vi "Teleop.vi"(0 "Call Context":T2, 1 "Match Info":T1={"Autonomous Elapsed Seconds"=0.0, "TeleOp Elapsed Seconds"=0.0, "Disabled Elapsed Seconds"=0.0, "Visited Autonomous"=FALSE, "Visited TeleOp"=FALSE, "Visited Disabled"=FALSE, "Autonomous Settings"={"Autonomous Style"=enum."Independent", "VI Refnum"=refnum}}) -> ()   [LabVIEW 2017]
doc: "This VI is called for each TeleOp packet received from the DS where the robot is not disabled. It is often used to read from the joysticks and update I/O or to update setpoints for timed control loops. It should complete and return within 20 milliseconds or it may miss DS packets."
uses:
  <vilib>/Rock Robotics/WPI/DriverStation/WPI_DriverStationDerivedRobotMode.ctl
  <vilib>/Rock Robotics/WPI/DriverStation/WPI_DriverStationMatch Info.ctl
  <vilib>/Rock Robotics/WPI/Utilities/WPI_GetSetVariantRefNum.vi
  <vilib>/Rock Robotics/Network Tables/NT Write Boolean Array.vi
  <vilib>/Rock Robotics/Network Tables/NT Write Numeric Array.vi
  <vilib>/Rock Robotics/Network Tables/NT Read Boolean.vi
  <vilib>/Rock Robotics/Network Tables/NT Read Number.vi
panel:
  out "Sample Slider 0":dbl(slide) scale=0.0..5.0
  out "Sample Boolean 1":bool
  out "Sample Boolean 0":bool
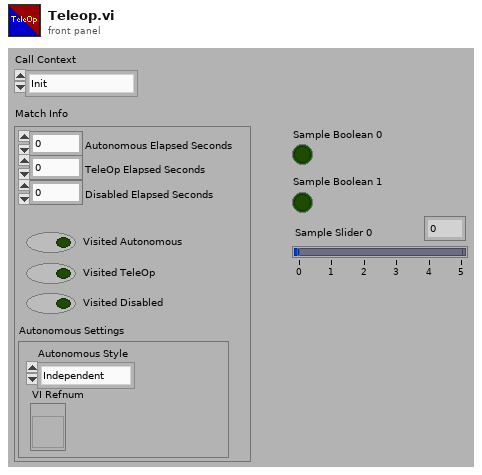
[diagram p1: front panel]
types:
  T1 = typedef "WPI_DriverStationMatch Info.ctl" = cluster{"Autonomous Elapsed Seconds":dbl, "TeleOp Elapsed Seconds":dbl, "Disabled Elapsed Seconds":dbl, "Visited Autonomous":bool, "Visited TeleOp":bool, "Visited Disabled":bool, "Autonomous Settings":cluster{"Autonomous Style":enum16{"Iterative", "Independent"}, "VI Refnum":refnum<vi>}}
  T2 = typedef "WPI_DriverStationDerivedRobotMode.ctl" = enum16{"Init", "Execute", "Stop"}
  T3 = typedef "WPI_JoystickDevRef.ctl" = cluster{"Device":T4}
  T4 = typedef "WPI_JoystickDeviceEnum.ctl" = enum16{"USB 0", "USB 1", "USB 2", "USB 3", "USB 4", "USB 5"}
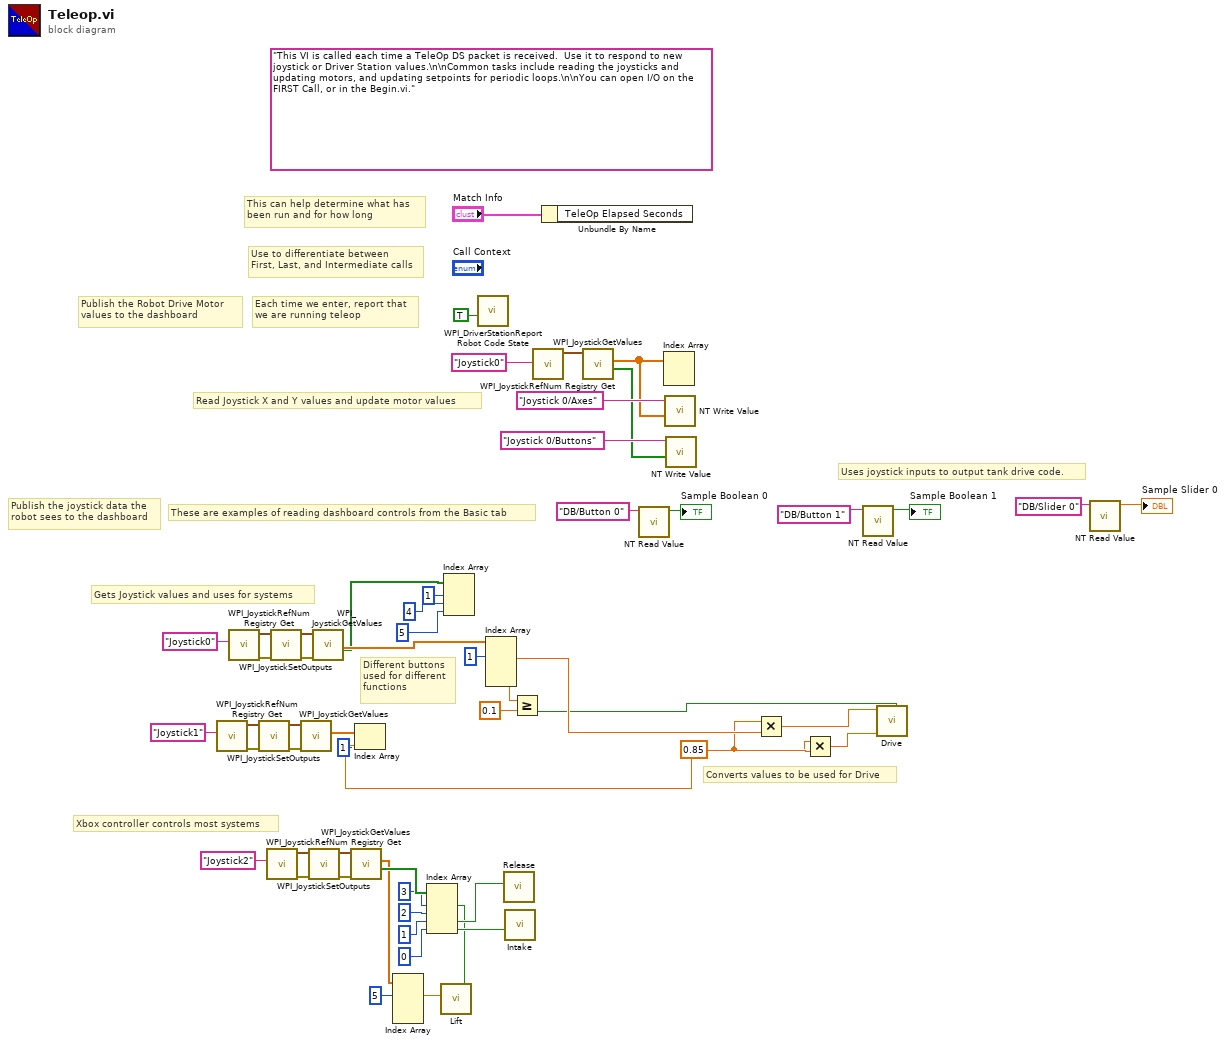
[diagram p0: block diagram]
diagram:
  w25 = 0.85
  (unwired) "This VI is called each time a TeleOp DS packet is received.  Use it to respond to new joystick or Driver Station values.\n\nCommon tasks include reading the joysticks and updating motors, and updating setpoints for periodic loops.\n\nYou can open I/O on the FIRST Call, or in the Begin.vi."
  # "Xbox controller controls most systems"
  # "Converts values to be used for Drive"
  # "Different buttons\nused for different\nfunctions"
  # "Gets Joystick values and uses for systems"
  # "Uses joystick inputs to output tank drive code."
  # "These are examples of reading dashboard controls from the Basic tab"
  # "Publish the Robot Drive Motor\nvalues to the dashboard"
  # "Publish the joystick data the\nrobot sees to the dashboard"
  # "Each time we enter, report that\nwe are running teleop"
  # "Use to differentiate between\nFirst, Last, and Intermediate calls"
  # "This can help determine what has\nbeen run and for how long"
  # "Read Joystick X and Y values and update motor values"
  n1 = call <vilib>:"WPI_JoystickRefNum Registry Get.vi"("refnum name"="Joystick1") -> ("error out"=w32:errorcluster, "JoystickDevRef"=w30:T3)  [unwired: 1 in, 8 out]
  n2 = call <vilib>:"WPI_JoystickRefNum Registry Get.vi"("refnum name"="Joystick0") -> ("error out"=w35:errorcluster, "JoystickDevRef"=w37:T3)  [unwired: 1 in, 8 out]
  n3 = call <vilib>:"WPI_JoystickSetOutputs.vi"("error in (no error)"=w32, "JoystickDevRef"=w30) -> ("error out"=w33:errorcluster, "JoystickDevRef"=w31:T3)  [unwired: 8 in]
  n4 = call <vilib>:"WPI_JoystickRefNum Registry Get.vi"("refnum name"="Joystick2") -> ("error out"=w15:errorcluster, "JoystickDevRef"=w17:T3)  [unwired: 1 in, 8 out]
  n5 = call <vilib>:"WPI_JoystickSetOutputs.vi"("error in (no error)"=w35, "JoystickDevRef"=w37) -> ("error out"=w34:errorcluster, "JoystickDevRef"=w36:T3)  [unwired: 8 in]
  n6 = call <vilib>:"WPI_JoystickGetValues.vi"("error in (no error)"=w33, "JoystickDevRef"=w31) -> ("Axes"=w28:dbl[])  [unwired: 5 in, 4 out]
  n7 = call <vilib>:"WPI_JoystickSetOutputs.vi"("error in (no error)"=w15, "JoystickDevRef"=w17) -> ("error out"=w14:errorcluster, "JoystickDevRef"=w16:T3)  [unwired: 8 in]
  n8 = call <vilib>:"WPI_JoystickGetValues.vi"("error in (no error)"=w34, "JoystickDevRef"=w36) -> ("Buttons"=w19:bool[], "Axes"=w42:dbl[])  [unwired: 5 in, 3 out]
  n9 = call <vilib>:"WPI_JoystickGetValues.vi"("error in (no error)"=w14, "JoystickDevRef"=w16) -> ("Buttons"=w13:bool[], "Axes"=w8:dbl[])  [unwired: 5 in, 3 out]
  n10 = Index Array(array=w28, index=1) -> (element=w26:dbl)
  n11 = Index Array(array=w8, index #1=5 ("index")) -> (element #1=w4:dbl)  [unwired: 3 in, 3 out]
  n12 = Index Array(array=w13, index #1=3 ("index"), index #2=2 ("index"), index #3=1 ("index"), index #4=0 ("index")) -> (element #1=w1:bool, element #3=w2:bool, element #4=w3:bool)  [unwired: 1 out]
  n13 = call "Lift.vi"("Half Effort"=w1, "Effort"=w4) -> ()  [unwired: 10 in]
  n14 = Index Array(array=w19, index #1=1 ("index"), index #2=4 ("index"), index #3=5 ("index")) -> ()  [unwired: 3 out]
  n15 = call <vilib>:"WPI_DriverStationReport Robot Code State.vi"("TeleOp"=TRUE ("Autonomous")) -> ()  [unwired: 10 in, 1 out]
  n16 = Index Array(array=w42, index #1=1 ("index")) -> (element #1=w27:dbl, element #3=w40:dbl)  [unwired: 3 in, 2 out]
  n17 = call "Release.vi"("Releasebuttonpressed?"=w2) -> ()  [unwired: 11 in]
  n18 = call "Intake.vi"("Intake?"=w3) -> ()  [unwired: 11 in]
  n19 = Greater Or Equal?(x=w40, y=0.1) -> (x >= y?=w22:bool)
  n20 = call <vilib>:"WPI_JoystickRefNum Registry Get.vi"("refnum name"="Joystick0") -> ("JoystickDevRef"=w54:T3)  [unwired: 1 in, 9 out]
  n21 = Unbundle By Name("Match Info") -> ()  [unwired: 1 out]
  n22 = call <vilib>:"WPI_JoystickGetValues.vi"("JoystickDevRef"=w54) -> ("Buttons"=w49:bool[], "Axes"=w50:dbl[])  [unwired: 6 in, 3 out]
  n23 = call-poly <vilib>:"NT Read Value.vi"("Name"="DB/Button 0" ("refnum name")) -> ("Boolean"=→"Sample Boolean 0":bool)  [unwired: 9 in, 1 out]
  n24 = Index Array(array=w50) -> ()  [unwired: 2 in, 2 out]
  n25 = call-poly <vilib>:"NT Write Value.vi"("Numeric Array"=w50, "Name"="Joystick 0/Axes") -> ()  [unwired: 9 in, 1 out]
  n26 = call-poly <vilib>:"NT Write Value.vi"("Boolean Array"=w49, "Name"="Joystick 0/Buttons") -> ()  [unwired: 9 in, 1 out]
  n27 = Multiply(x=w25, y=w27) -> (x*y=w24:dbl)
  n28 = Multiply(x=w25, y=w26) -> (x*y=w23:dbl)
  n29 = call-poly <vilib>:"NT Read Value.vi"("Name"="DB/Button 1" ("refnum name")) -> ("Boolean"=→"Sample Boolean 1":bool)  [unwired: 9 in, 1 out]
  n30 = call "Drive.vi"("Slow?"=w22, "Drive R"=w23, "Drive L"=w24) -> ()  [unwired: 9 in]
  n31 = call-poly <vilib>:"NT Read Value.vi"("Name"="DB/Slider 0" ("refnum name")) -> ("Numeric"=→"Sample Slider 0":dbl)  [unwired: 9 in, 1 out]
